vi "ADAM6018.vi"(11 "Remote IP Address 2":string="192.168.0.165") -> (0 "Array":sgl[](array[numeric])=[26.245518, 23.964294, 29.78561, 24.086367])   [LabVIEW 2012]
uses:
  nimodbus121/nimodbus121/71/vi.lib/NI Modbus.llb/MB Modbus Command.ctl
panel:
  out "Slave Input Registers 2":u16[](array[numeric])=[16547, 16248, 17011, 16264] caption="Slave Input Registers (Read Only)"
  in  "Modbus Command":T1={"Function Code"=4, "Starting Address"=0, "Quantity"=4, "Data"=[], "Discrete"=[]} {"Function Code" items=["Read Coils"=1, "Read Discrete Inputs"=2, "Read Holding Registers"=3, "Read Input Registers"=4, "Write Single Coil"=5, "Write Single Register"=6, "Read Exception Status"=7, "Write Multiple Coils"=15, "Write Multiple Registers"=16]}
  out "error out":errorcluster
  in  "Remote Port 2":u16=502
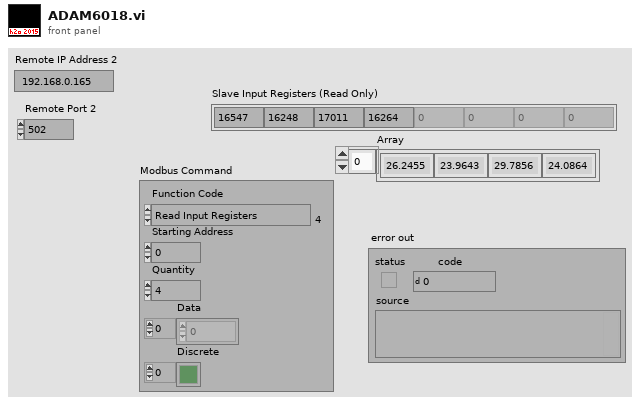
[diagram p1: front panel]
types:
  T1 = typedef "MB Modbus Command.ctl" = cluster{"Function Code":u8, "Starting Address":u16, "Quantity":u16, "Data":u16[], "Discrete":bool[]}
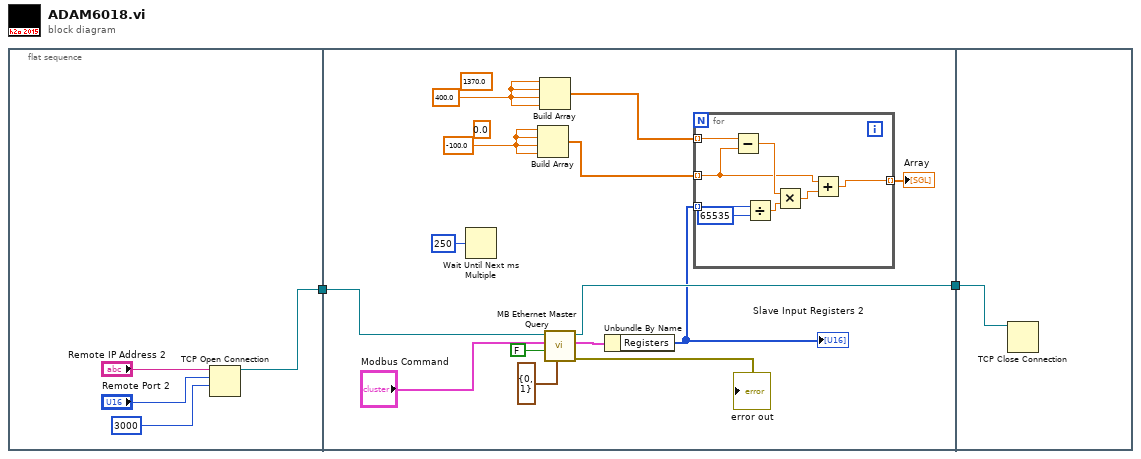
[diagram p0: block diagram]
diagram:
  n1 = flat-sequence {
    tunnel: [w3] -> w1
    tunnel: [w14] -> w2
    tunnel: w1 -> [w13]
    tunnel: w2 -> [w29]
    frame #0 {
      n2 = TCP Open Connection(address="Remote IP Address 2", remote port or service name="Remote Port 2", timeout ms (60000)=3000) -> (connection ID=w3:refnum<k5>)  [unwired: 2 in, 1 out]
    }
    frame #1 {
      w8 = 400.0 ("element")
      (unwired) 1370.0 ("element")
      w7 = -100.0 ("element")
      (unwired) 0.0 ("element")
      n3 = Wait Until Next ms Multiple(millisecond multiple=u32 250) -> ()  [unwired: 1 out]
      n4 = Build Array(w7, w7, w7, w7) -> (w11:dbl[])
      n5 = Build Array(w8, w8, w8, w8) -> (w9:dbl[])
      n6 = call "MB Ethernet Master Query.vi"("MBAP Header"=cluster{"Transaction ID":u16, "Unit ID":u8} {"Transaction ID"=0, "Unit ID"=1}, "Use MODBUS Data Unit?"=FALSE, "Modbus Command"="Modbus Command", "TCP Connection Refnum in"=w13) -> ("error out"=→"error out":errorcluster, "Registers"=w16:cluster{"Registers":u16[], "Discrete":bool[]}, "TCP Connection Refnum (dup)"=w14:refnum<k5>)  [unwired: 3 in, 2 out]
      n7 = Unbundle By Name(w16) -> ("Registers"=w10:u16[])
      "Slave Input Registers 2" <- w10
      n8 = for {
        tunnel: [w22] -> w12 mode=indexing
        tunnel: w11 -> [w21] mode=indexing
        tunnel: w10 -> [w28] mode=indexing
        tunnel: w9 -> [w23] mode=indexing
        n9 = Subtract(x=w23, y=w21) -> (x-y=w25:dbl)
        n10 = Divide(x=w28, y=u16 65535) -> (x/y=w26:dbl)
        n11 = Multiply(x=w25, y=w26) -> (x*y=w24:dbl)
        n12 = Add(x=w21, y=w24) -> (x+y=w22:dbl)
      }
      "Array" <- w12
    }
    frame #2 {
      n13 = TCP Close Connection(connection ID=w29) -> ()  [unwired: 2 in, 2 out]
    }
  }
